vi "InitIMU.vi"() -> (0 "error out":errorcluster, 3 "I2C Ref Out":T1)   [LabVIEW 2016]
uses:
  <vilib>/myRIO/Instrument Drivers/Onboard IO/I2C/typedefs/I2C Transfer Rate.ctl
  <vilib>/myRIO/Instrument Drivers/Onboard IO/I2C/I2C.lvlib
  <vilib>/myRIO/Instrument Drivers/Onboard IO/I2C/typedefs/I2C Configuration.ctl
  <vilib>/myRIO/Common/Instrument Driver Framework/myRIO v1.0/I2C/typedefs/I2C Channels Enum.ctl
  <vilib>/myRIO/Common/Instrument Driver Framework/Utilities/typedefs/Generic FPGA Reference.ctl
  <vilib>/myRIO/Common/Instrument Driver Framework/Utilities/typedefs/myRIO v1.0 Reference.ctl
  <vilib>/myRIO/Common/Instrument Driver Framework/Utilities/typedefs/Hardware Version Enum.ctl
  <vilib>/myRIO/Common/Instrument Driver Framework/Utilities/typedefs/myRIO Generic Hardware Reference.ctl
  <vilib>/myRIO/Instrument Drivers/Onboard IO/I2C/typedefs/I2C Reference.ctl
  <vilib>/userdefined/High Color/nirio_resource_hc.ctl
  <vilib>/myRIO/Common/Instrument Driver Framework/myRIO v1.0/I2C/vis/myRIO v1.1 Open I2C.vi
  <vilib>/myRIO/Instrument Drivers/Onboard IO/I2C/vis/myRIO I2C Open.xnode
  <vilib>/myRIO/Instrument Drivers/Onboard IO/I2C/typedefs/I2C User Configuration.ctl
  LIFA MPU-60X0 LV9/RegisterAddresses.ctl
  LIFA MPU-60X0 LV9/LIFA MPU-60X0.lvlib
panel:
  out "x != y?":bool
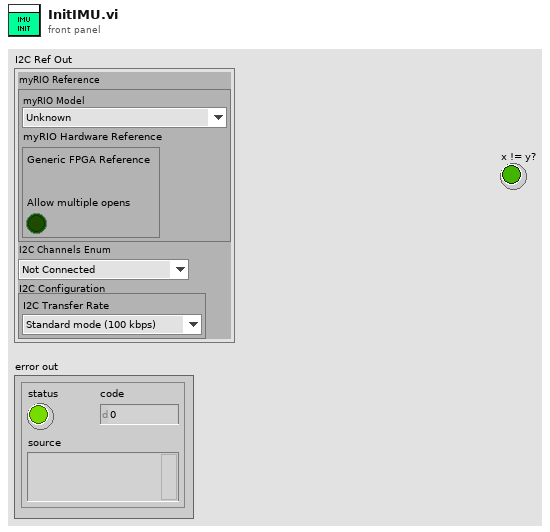
[diagram p1: front panel]
types:
  T1 = typedef "I2C.lvlib/I2C Reference.ctl" = cluster{"myRIO Reference":T2, "I2C Channels Enum":T6, "I2C Configuration":T7}
  T2 = typedef "myRIO Generic Hardware Reference.ctl" = cluster{"myRIO Model":T3, "myRIO Hardware Reference":T4}
  T3 = typedef "Hardware Version Enum.ctl" = enum16{"Unknown", "myRIO-1900", "myRIO-1950", "roboRIO", "NI ELVIS RIO CM"}
  T4 = typedef "myRIO v1.0 Reference.ctl" = cluster{"Generic FPGA Reference":T5, "Allow multiple opens":bool}
  T5 = typedef "Generic FPGA Reference.ctl" = refnum<k20>
  T6 = typedef "I2C Channels Enum.ctl" = enum16{"Not Connected", "A/I2C", "B/I2C", "I2C/I2C"}
  T7 = typedef "I2C.lvlib/I2C Configuration.ctl" = cluster{"I2C Transfer Rate":T8}
  T8 = typedef "I2C.lvlib/I2C Transfer Rate.ctl" = enum16{"Standard mode (100 kbps)", "Fast mode (400 kbps)"}
  T9 = typedef "LIFA MPU-60X0.lvlib/RegisterAddresses.ctl" = u16
  T10 = cluster{"length":u8, "bitStart":u8, "data":u8, "Register Addresses":T9}
  T11 = typedef "I2C.lvlib/I2C User Configuration.ctl" = cluster{"I2C Transfer Rate":T8}
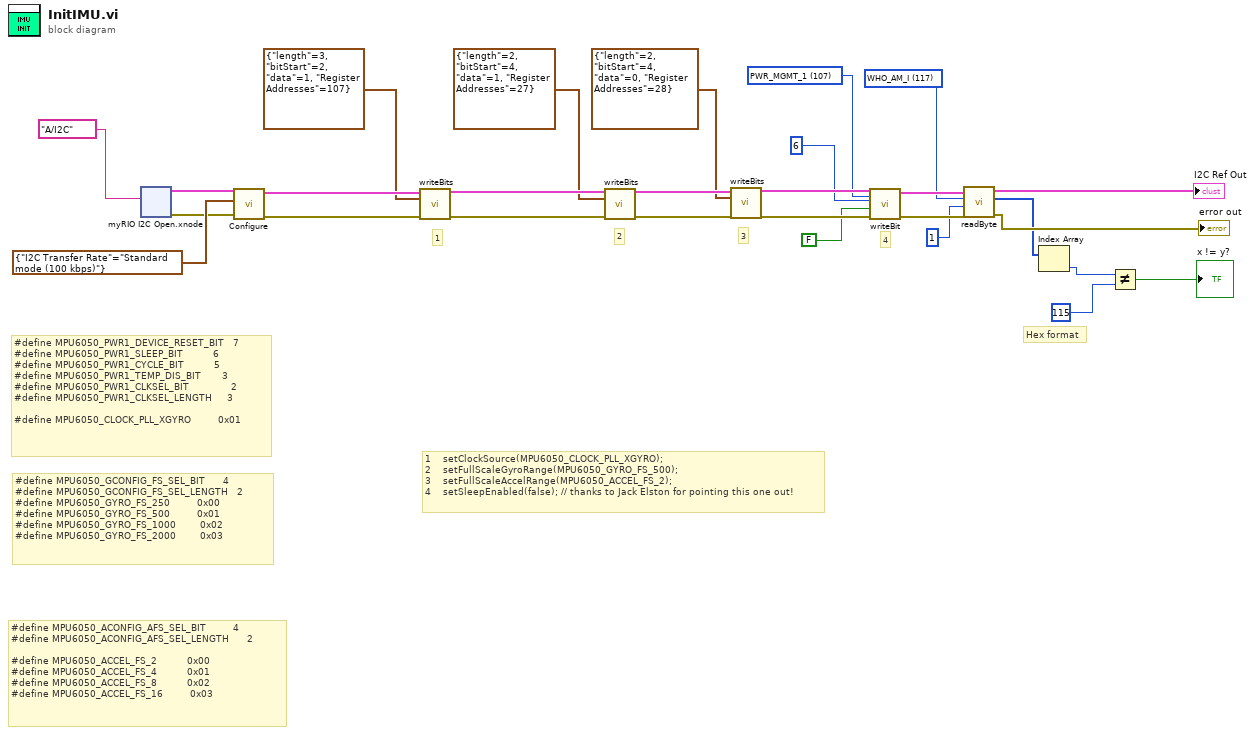
[diagram p0: block diagram]
diagram:
  w6 = T9 117 items=["SELF_TEST_X"=13, "SELF_TEST_Y"=14, "SELF_TEST_Z"=15, "SELF_TEST_A"=16, "SMPLRT_DIV"=25, "CONFIG"=26, "GYRO_CONFIG"=27, "ACCEL_CONFIG"=28, "MOT_THR"=31, "FIFO_EN"=35, "I2C_MST_CTRL"=36, "I2C_SLV0_ADDR"=37, "I2C_SLV0_REG"=38, "I2C_SLV0_CTRL"=39, "I2C_SLV1_ADDR"=40, "I2C_SLV1_REG"=41, "I2C_SLV1_CTRL"=42, "I2C_SLV2_ADDR"=43, "I2C_SLV2_REG"=44, "I2C_SLV2_CTRL"=45, "I2C_SLV3_ADDR"=46, "I2C_SLV3_REG"=47, "I2C_SLV3_CTRL"=48, "I2C_SLV4_ADDR"=49, "I2C_SLV4_REG"=50, "I2C_SLV4_DO"=51, "I2C_SLV4_CTRL"=52, "I2C_SLV4_DI"=53, "I2C_MST_STATUS"=54, "INT_PIN_CFG"=55, "INT_ENABLE"=56, "INT_STATUS"=58, "ACCEL_XOUT_H"=59, "ACCEL_XOUT_L"=60, "ACCEL_YOUT_H"=61, "ACCEL_YOUT_L"=62, "ACCEL_ZOUT_H"=63, "ACCEL_ZOUT_L"=64, "TEMP_OUT_H"=65, "TEMP_OUT_L"=66, "GYRO_XOUT_H"=67, "GYRO_XOUT_L"=68, "GYRO_YOUT_H"=69, "GYRO_YOUT_L"=70, "GYRO_ZOUT_H"=71, "GYRO_ZOUT_L"=72, "EXT_SENS_DATA_00"=73, "EXT_SENS_DATA_01"=74, "EXT_SENS_DATA_02"=75, "EXT_SENS_DATA_03"=76, "EXT_SENS_DATA_04"=77, "EXT_SENS_DATA_05"=78, "EXT_SENS_DATA_06"=79, "EXT_SENS_DATA_07"=80, "EXT_SENS_DATA_08"=81, "EXT_SENS_DATA_09"=82, "EXT_SENS_DATA_10"=83, "EXT_SENS_DATA_11"=84, "EXT_SENS_DATA_12"=85, "EXT_SENS_DATA_13"=86, "EXT_SENS_DATA_14"=87, "EXT_SENS_DATA_15"=88, "EXT_SENS_DATA_16"=89, "EXT_SENS_DATA_17"=90, "EXT_SENS_DATA_18"=91, "EXT_SENS_DATA_19"=92, "EXT_SENS_DATA_20"=93, "EXT_SENS_DATA_21"=94, "EXT_SENS_DATA_22"=95, "EXT_SENS_DATA_23"=96, "I2C_SLV0_DO"=99, "I2C_SLV1_DO"=100, "I2C_SLV2_DO"=101, "I2C_SLV3_DO"=102, "I2C_MST_DELAY_CTRL"=103, "SIGNAL_PATH_RESET"=104, "MOT_DETECT_CTRL"=105, "USER_CTRL"=106, "PWR_MGMT_1"=107, "PWR_MGMT_2"=108, "FIFO_COUNTH"=114, "FIFO_COUNTL"=115, "FIFO_R_W"=116, "WHO_AM_I"=117] ("Register Addresses")
  w13 = T9 107 items=["SELF_TEST_X"=13, "SELF_TEST_Y"=14, "SELF_TEST_Z"=15, "SELF_TEST_A"=16, "SMPLRT_DIV"=25, "CONFIG"=26, "GYRO_CONFIG"=27, "ACCEL_CONFIG"=28, "MOT_THR"=31, "FIFO_EN"=35, "I2C_MST_CTRL"=36, "I2C_SLV0_ADDR"=37, "I2C_SLV0_REG"=38, "I2C_SLV0_CTRL"=39, "I2C_SLV1_ADDR"=40, "I2C_SLV1_REG"=41, "I2C_SLV1_CTRL"=42, "I2C_SLV2_ADDR"=43, "I2C_SLV2_REG"=44, "I2C_SLV2_CTRL"=45, "I2C_SLV3_ADDR"=46, "I2C_SLV3_REG"=47, "I2C_SLV3_CTRL"=48, "I2C_SLV4_ADDR"=49, "I2C_SLV4_REG"=50, "I2C_SLV4_DO"=51, "I2C_SLV4_CTRL"=52, "I2C_SLV4_DI"=53, "I2C_MST_STATUS"=54, "INT_PIN_CFG"=55, "INT_ENABLE"=56, "INT_STATUS"=58, "ACCEL_XOUT_H"=59, "ACCEL_XOUT_L"=60, "ACCEL_YOUT_H"=61, "ACCEL_YOUT_L"=62, "ACCEL_ZOUT_H"=63, "ACCEL_ZOUT_L"=64, "TEMP_OUT_H"=65, "TEMP_OUT_L"=66, "GYRO_XOUT_H"=67, "GYRO_XOUT_L"=68, "GYRO_YOUT_H"=69, "GYRO_YOUT_L"=70, "GYRO_ZOUT_H"=71, "GYRO_ZOUT_L"=72, "EXT_SENS_DATA_00"=73, "EXT_SENS_DATA_01"=74, "EXT_SENS_DATA_02"=75, "EXT_SENS_DATA_03"=76, "EXT_SENS_DATA_04"=77, "EXT_SENS_DATA_05"=78, "EXT_SENS_DATA_06"=79, "EXT_SENS_DATA_07"=80, "EXT_SENS_DATA_08"=81, "EXT_SENS_DATA_09"=82, "EXT_SENS_DATA_10"=83, "EXT_SENS_DATA_11"=84, "EXT_SENS_DATA_12"=85, "EXT_SENS_DATA_13"=86, "EXT_SENS_DATA_14"=87, "EXT_SENS_DATA_15"=88, "EXT_SENS_DATA_16"=89, "EXT_SENS_DATA_17"=90, "EXT_SENS_DATA_18"=91, "EXT_SENS_DATA_19"=92, "EXT_SENS_DATA_20"=93, "EXT_SENS_DATA_21"=94, "EXT_SENS_DATA_22"=95, "EXT_SENS_DATA_23"=96, "I2C_SLV0_DO"=99, "I2C_SLV1_DO"=100, "I2C_SLV2_DO"=101, "I2C_SLV3_DO"=102, "I2C_MST_DELAY_CTRL"=103, "SIGNAL_PATH_RESET"=104, "MOT_DETECT_CTRL"=105, "USER_CTRL"=106, "PWR_MGMT_1"=107, "PWR_MGMT_2"=108, "FIFO_COUNTH"=114, "FIFO_COUNTL"=115, "FIFO_R_W"=116, "WHO_AM_I"=117] ("Register Addresses")
  # "Hex format"
  # "4"
  # "3"
  # "#define MPU6050_ACONFIG_AFS_SEL_BIT         4\n#define MPU6050_ACONFIG_AFS_SEL_LENGTH      2\n\n#define MPU6050_ACCEL_FS_2          0x00\n#define MPU6050_ACCEL_FS_4          0x01\n#define MPU6050_ACCEL_FS_8          0x02\n#define MPU6050_ACCEL_FS_16         0x03"
  # "2"
  # "#define MPU6050_GCONFIG_FS_SEL_BIT      4\n#define MPU6050_GCONFIG_FS_SEL_LENGTH   2\n#define MPU6050_GYRO_FS_250         0x00\n#define MPU6050_GYRO_FS_500         0x01\n#define MPU6050_GYRO_FS_1000        0x02\n#define MPU6050_GYRO_FS_2000        0x03"
  # "1"
  # "1    setClockSource(MPU6050_CLOCK_PLL_XGYRO);\n2    setFullScaleGyroRange(MPU6050_GYRO_FS_500);\n3    setFullScaleAccelRange(MPU6050_ACCEL_FS_2);\n4    setSleepEnabled(false); // thanks to Jack Elston for pointing this one out!"
  # "#define MPU6050_PWR1_DEVICE_RESET_BIT   7\n#define MPU6050_PWR1_SLEEP_BIT          6\n#define MPU6050_PWR1_CYCLE_BIT          5\n#define MPU6050_PWR1_TEMP_DIS_BIT       3\n#define MPU6050_PWR1_CLKSEL_BIT              2\n#define MPU6050_PWR1_CLKSEL_LENGTH     3\n\n#define MPU6050_CLOCK_PLL_XGYRO         0x01"
  n1 = xnode "myRIO I2C Open.xnode"("Channel Name"=tag "A/I2C") -> ("error out"=w27:errorcluster, "I2C Ref Out"=w26:T1)  [unwired: 2 in]
  n2 = call <vilib>:"Configure.vi"("error in (no error)"=w27, "I2C User Configuration"=T11 {"I2C Transfer Rate"=enum."Standard mode (100 kbps)"}, "I2C Ref In"=w26) -> ("error out"=w24:errorcluster, "I2C Ref Out"=w23:T1)  [unwired: 7 in]
  n3 = call "writeBits.vi"("I2C Ref Out"=w23, "Params"=T10 {"length"=3, "bitStart"=2, "data"=1, "Register Addresses"=107}, "error in (no error)"=w24) -> ("I2C Ref Out 2"=w21:T1, "error out"=w20:errorcluster)  [unwired: 11 in]
  n4 = call "writeBits.vi"("I2C Ref Out"=w21, "Params"=T10 {"length"=2, "bitStart"=4, "data"=1, "Register Addresses"=27}, "error in (no error)"=w20) -> ("I2C Ref Out 2"=w18:T1, "error out"=w17:errorcluster)  [unwired: 11 in]
  n5 = call "writeBits.vi"("I2C Ref Out"=w18, "Params"=T10 {"length"=2, "bitStart"=4, "data"=0, "Register Addresses"=28}, "error in (no error)"=w17) -> ("I2C Ref Out 2"=w15:T1, "error out"=w14:errorcluster)  [unwired: 11 in]
  n6 = call "writeBit.vi"("Register Addresses"=w13, "error in (no error)"=w14, "Enable/Disable"=FALSE, "bitNum"=u8 6, "I2C Ref In"=w15) -> ("error out"=w9:errorcluster, "I2C Ref Out"=w10:T1)  [unwired: 5 in]
  n7 = call "readByte.vi"("error in (no error)"=w9, "Byte Count"=u32 1, "Register Addresses"=w6, "I2C Ref In"=w10) -> ("error out"=→"error out":errorcluster, "Bytes Read"=w4:u8[], "I2C Ref Out"=→"I2C Ref Out":T1)  [unwired: 5 in]
  n8 = Index Array(array=w4) -> (element=w3:u8)  [unwired: 1 in]
  n9 = Not Equal?(x=w3, y=u8 115) -> (x != y?=→"x != y?":bool)
